vi "Update Dependency.vi"(6 "Level":string, 8 "error in (no error)":errorcluster, 9 "owned":bool, 10 "SMO":refnum<class "SMO.lvclass">, 11 "Attribute.Dependencies in":refnum<class "Attribute.Dependencies.lvclass">) -> (0 "error out":errorcluster, 3 "Attribute.Dependencies out":refnum<class "Attribute.Dependencies.lvclass">)   [LabVIEW 2021, in "smo.lvlib" / "Attribute.Dependencies.lvclass"]
uses:
  Attribute.Dependencies.lvclass
  SMO/SMO.lvclass
  DependencyAttr--Cluster.ctl
  Attribute.Dependencies.lvclass/Attribute.Dependencies.ctl
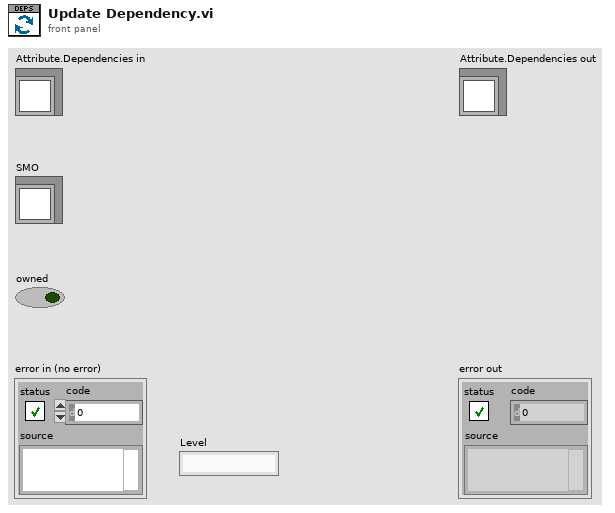
[diagram p1: front panel]
types:
  T1 = typedef "smo.lvlib/Attribute.Dependencies.lvclass/DependencyAttr--Cluster.ctl" = cluster{"Name":string, "GUID":string, "owned":bool, "shared":bool, "Level":string, "SMO":refnum<class "SMO.lvclass">}
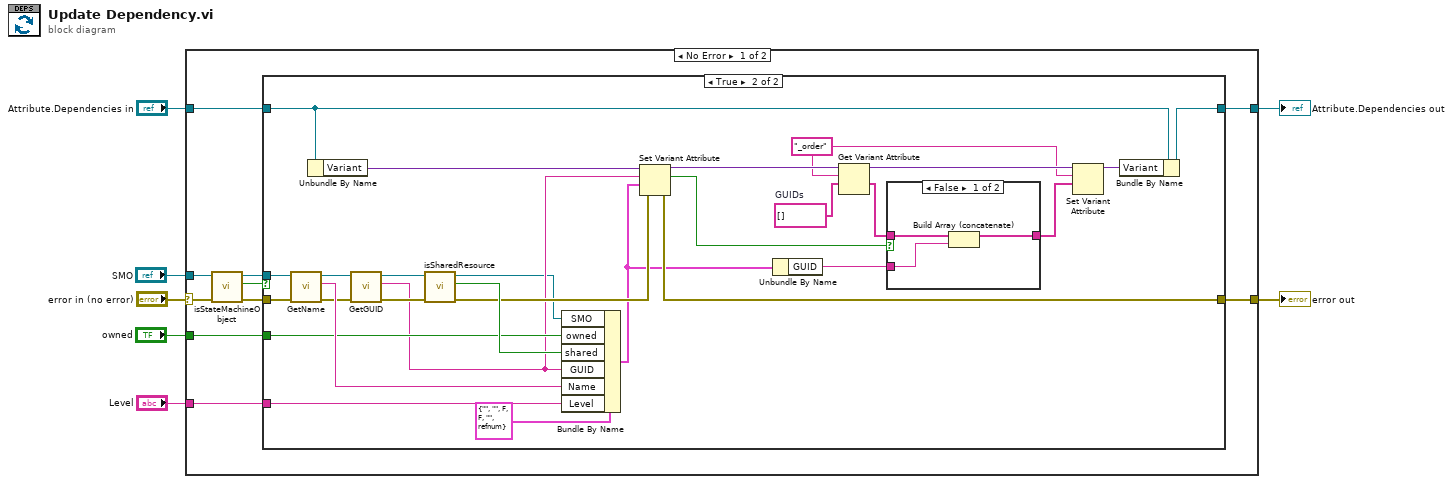
[diagram p0: block diagram]
diagram:
  n1 = case shown="No Error" "error in (no error)" {
    selector: "error in (no error)" -> [w11 w53]
    tunnel: [w10 w53] -> w6
    tunnel: [w17 w52] -> w4
    tunnel: "Attribute.Dependencies in" -> [w16 w52]
    tunnel: "SMO" -> [w15 _]
    tunnel: "owned" -> [w9 _]
    tunnel: "Level" -> [w8 _]
    frame No Error {
      n2 = call "isStateMachineObject.vi"("error in (no error)"=w11, "SMO"=w15) -> ("error out"=w12:errorcluster, "is SMO?"=w13:bool, "SMO out"=w14:refnum<class "SMO.lvclass">)  [unwired: 7 in]
      n3 = case shown="True" w13 {
        tunnel: [w19 w42] -> w17
        tunnel: w16 -> [w19 w41]
        tunnel: w14 -> [_ w37]
        tunnel: w12 -> [w18 w36]
        tunnel: [w18 w34] -> w10
        tunnel: w9 -> [_ w33]
        tunnel: w8 -> [_ w31]
        frame False {
        }
        frame True {
          w28 = string[] []  # GUIDs
          w25 = "_order" ("Attribute Name")
          n4 = call "GetName.vi"("error in (no error)"=w36, "SMO"=w37) -> ("error out"=w39:errorcluster, "Name"=w43:string, "SMO out"=w47:refnum<class "SMO.lvclass">)  [unwired: 6 in, 1 out]
          n5 = Unbundle By Name(w41) -> ("Variant"=w40:variant)
          n6 = call "GetGUID.vi"("error in (no error)"=w39, "SMO"=w47) -> ("error out"=w38:errorcluster, "GUID"=w32:string, "SMO out"=w46:refnum<class "SMO.lvclass">)  [unwired: 7 in]
          n7 = call "isSharedResource.vi"("error in (no error)"=w38, "SMO in"=w46) -> ("error out"=w35:errorcluster, "shared resource"=w44:bool, "SMO out"=w30:refnum<class "SMO.lvclass">)  [unwired: 7 in]
          n8 = Bundle By Name(cluster=T1 {"Name"="", "GUID"="", "owned"=FALSE, "shared"=FALSE, "Level"="", "SMO"=refnum} ("Dependency"), "SMO"=w30, "owned"=w33, "shared"=w44, "GUID"=w32, "Name"=w43, "Level"=w31) -> (w22:T1)
          n9 = Set Variant Attribute(Variant=w40, name=w32, value=w22, error in=w35) -> (Variant out=w29:variant, replaced=w24:bool, error out=w34:errorcluster)
          n10 = Unbundle By Name(w22) -> ("GUID"=w21:string)
          n11 = Get Variant Attribute(Variant=w29, name=w25, default value (empty Variant)=w28) -> (duplicate Variant=w26:variant, value=w23:string[])  [unwired: 1 in, 2 out]
          n12 = case shown="False" w24 {
            tunnel: w23 -> [w50 w51]
            tunnel: w21 -> [w49 _]
            tunnel: [w48 w51] -> w20
            frame False {
              n13 = Build Array (concatenate)(w50, w49) -> (w48:string[])
            }
            frame True {
            }
          }
          n14 = Set Variant Attribute(Variant=w26, name=w25, value=w20) -> (Variant out=w27:variant)  [unwired: 1 in, 2 out]
          n15 = Bundle By Name(cluster=w41, "Variant"=w27) -> (w42:refnum<class "Attribute.Dependencies.lvclass">)
        }
      }
    }
    frame Error {
    }
  }
  "error out" <- w6
  "Attribute.Dependencies out" <- w4
